vi "Read Status.vi"(8 "error in":errorcluster, 11 "CoreOOB_Tx in":refnum<class "CIFTemplateCoreOOB_Tx.lvclass">) -> (0 "error out":errorcluster, 2 "Status":T1 {"Monitor Doubles"."4" format="%#_9g"; "Monitor Doubles"."3" format="%#_9g"; "Monitor Doubles"."2" format="%#_9g"; "Monitor Doubles"."1" format="%#_9g"}, 3 "CoreOOB_Tx out":refnum<class "CIFTemplateCoreOOB_Tx.lvclass">)   [LabVIEW 2021, in "CIFTemplateCoreOOB_Tx.lvclass"]
uses:
  CIFTemplateCoreOOB_Tx.lvclass
  CIFTemplateCoreOOB_Tx.lvclass/CIFTemplateCoreOOB_Tx.ctl
  CIFTemplateCommon/Typedef/Simple Error.ctl
  CIFTemplateCommon/CIFTemplateCommon.lvlib
  CIFTemplateCommon/Typedef/Plugin State.ctl
  CIFTemplateCommon/Typedef/Plugin Status.ctl
  CIFTemplateCommon/Typedef/Timing Stats Base.ctl
  CIFTemplateCommon/Typedef/Timing Statistics.ctl
  CIFTemplateCommon/Typedef/FIFO Statistics.ctl
  CIFTemplateCommon/Typedef/Monitor Doubles.ctl
  CIFTemplateCommon/Typedef/Monitor U64.ctl
  CIFTemplateCommon/Typedef/Monitor I64.ctl
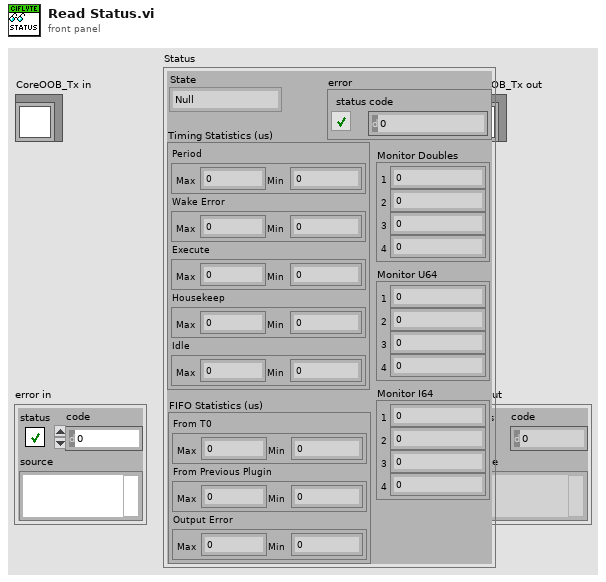
[diagram p1: front panel]
types:
  T1 = typedef "CIFTemplateCommon.lvlib/Plugin Status.ctl" = cluster{"State":T2, "Timing Statistics (us)":T3, "FIFO Statistics (us)":T5, "error":T6, "Monitor Doubles":T7, "Monitor U64":T8, "Monitor I64":T9}
  T2 = typedef "CIFTemplateCommon.lvlib/Plugin State.ctl" = enum32{"Null", "Creating", "Listening", "Running", "CleaningUp", "Destroying"}
  T3 = typedef "CIFTemplateCommon.lvlib/Timing Statistics.ctl" = cluster{"Period":T4, "Wake Error":T4, "Execute":T4, "Housekeep":T4, "Idle":T4}
  T4 = typedef "CIFTemplateCommon.lvlib/Timing Stats Base.ctl" = cluster{"Max":i32, "Min":i32}
  T5 = typedef "CIFTemplateCommon.lvlib/FIFO Statistics.ctl" = cluster{"From T0":T4, "From Previous Plugin":T4, "Output Error":T4}
  T6 = typedef "CIFTemplateCommon.lvlib/Simple Error.ctl" = cluster{"status":bool, "code":i32}
  T7 = typedef "CIFTemplateCommon.lvlib/Monitor Doubles.ctl" = cluster{"1":dbl, "2":dbl, "3":dbl, "4":dbl}
  T8 = typedef "CIFTemplateCommon.lvlib/Monitor U64.ctl" = cluster{"1":u64, "2":u64, "3":u64, "4":u64}
  T9 = typedef "CIFTemplateCommon.lvlib/Monitor I64.ctl" = cluster{"1":i64, "2":i64, "3":i64, "4":i64}
  T10 = typedef "CIFTemplateCoreOOB_Tx.lvclass/Template Payload.ctl" = cluster{"Status":T1, "Plugin Overrides":T11}
  T11 = typedef "CIFTemplateCommon.lvlib/Plugin Overrides.ctl" = cluster{"Timing Overrides":T12}
  T12 = typedef "CIFTemplateCommon.lvlib/Timing Overrides.ctl" = cluster{"Override Timing":bool, "Period (s)":dbl}
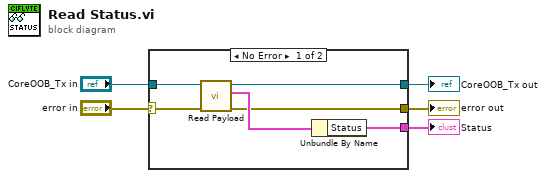
[diagram p0: block diagram]
diagram:
  n1 = case shown="No Error" "error in" {
    selector: "error in" -> [w7 w12]
    tunnel: [w6 w12] -> w4
    tunnel: [w10 w13] -> w2
    tunnel: "CoreOOB_Tx in" -> [w11 w13]
    tunnel: [w8 _] -> w1
    frame No Error {
      n2 = call "Read Payload.vi"("error in"=w7, "CoreOOB_Tx in"=w11) -> ("error out"=w6:errorcluster, "data"=w9:T10, "CoreOOB_Tx out"=w10:refnum<class "CIFTemplateCoreOOB_Tx.lvclass">)  [unwired: 7 in]
      n3 = Unbundle By Name(w9) -> ("Status"=w8:T1)
    }
    frame Error {
    }
  }
  "error out" <- w4
  "CoreOOB_Tx out" <- w2
  "Status" <- w1
